vi "Check for End of Output Sweep.vi"(8 "error in (no error)":errorcluster, 10 "current generation level":dbl, 11 "regaultion settings":T1) -> (0 "error out":errorcluster, 2 "generation level":dbl, 3 "sweep done":bool)   [LabVIEW 2021]
uses:
  controls/regulation target.ctl
  controls/regulation target value units.ctl
  controls/regulation settings.ctl
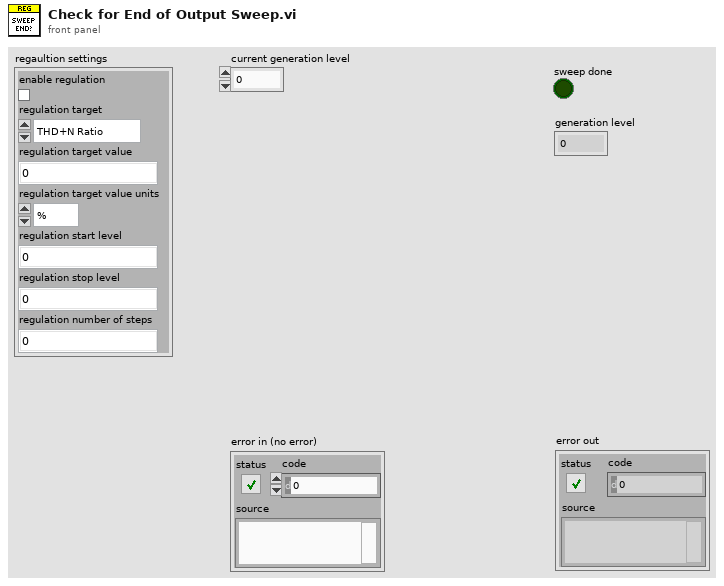
[diagram p1: front panel]
types:
  T1 = typedef "regulation settings.ctl" = cluster{"enable regulation":bool, "regulation target":T2, "regulation target value":dbl, "regulation target value units":T3, "regulation start level":dbl, "regulation stop level":dbl, "regulation number of steps":u32}
  T2 = typedef "regulation target.ctl" = enum32{"THD+N Ratio", "Output Power"}
  T3 = typedef "regulation target value units.ctl" = enum32{"%", "W"}
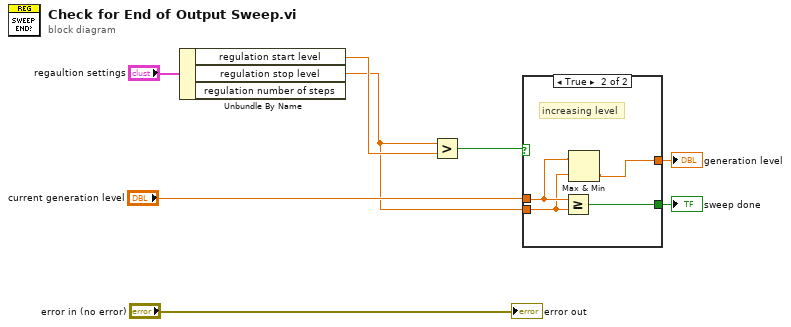
[diagram p0: block diagram]
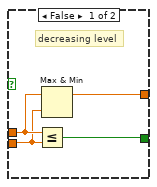
[diagram p2: hidden frame]
diagram:
  n1 = Unbundle By Name("regaultion settings") -> ("regulation start level"=w5:dbl, "regulation stop level"=w3:dbl)  [unwired: 1 out]
  n2 = Greater?(x=w3, y=w5) -> (0:w4:bool)
  n3 = case shown="True" w4 {
    tunnel: "current generation level" -> [w11 w15]
    tunnel: w3 -> [w10 w14]
    tunnel: [w12 w16] -> w2
    tunnel: [w9 w13] -> w1
    frame False {
      # "decreasing level"
      n4 = Less Or Equal?(x=w11, y=w10) -> (x <= y?=w12:bool)
      n5 = Max & Min(x=w11, y=w10) -> (max(x,y)=w9:dbl)  [unwired: 1 out]
    }
    frame True {
      # "increasing level"
      n6 = Greater Or Equal?(x=w15, y=w14) -> (x >= y?=w16:bool)
      n7 = Max & Min(x=w15, y=w14) -> (min(x,y)=w13:dbl)  [unwired: 1 out]
    }
  }
  "sweep done" <- w2
  "generation level" <- w1
  "error out" <- "error in (no error)"
